vi "traffic lights using parallelism.vi"() -> ()   [LabVIEW 2018]
panel:
  out "GREEN":bool
  out "YELLOW":bool
  out "RED":bool
  out "7 2":bool
  out "6 2":bool
  out "5 2":bool
  out "4 2":bool
  out "3 2":bool
  out "2 2":bool
  out "1 2":bool
  out "7":bool
  out "6":bool
  out "5":bool
  out "4":bool
  out "3":bool
  out "2":bool
  out "1":bool
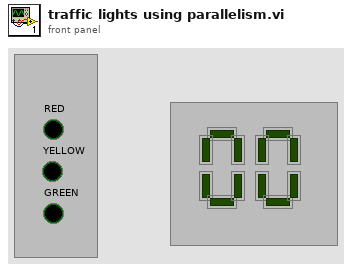
[diagram p1: front panel]
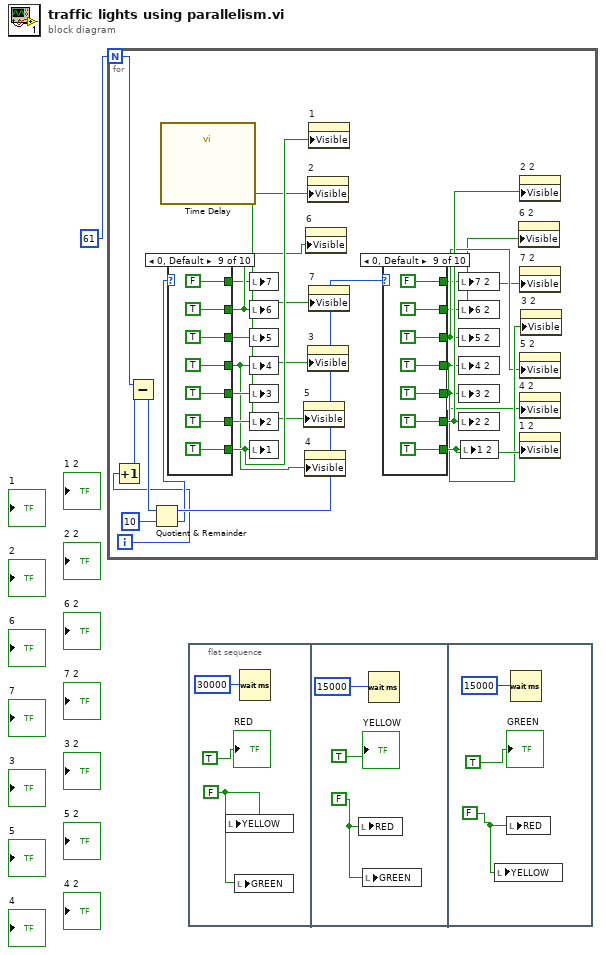
[diagram p0: block diagram]
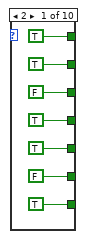
[diagram p2: hidden frame]
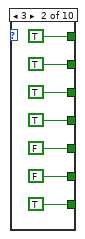
[diagram p3: hidden frame]
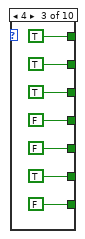
[diagram p4: hidden frame]
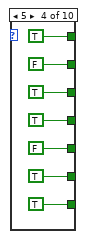
[diagram p5: hidden frame]
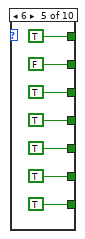
[diagram p6: hidden frame]
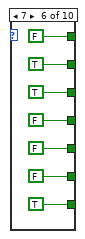
[diagram p7: hidden frame]
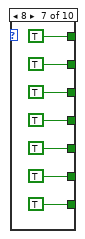
[diagram p8: hidden frame]
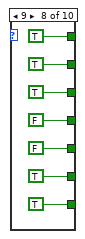
[diagram p9: hidden frame]
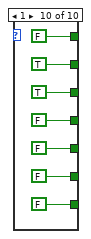
[diagram p10: hidden frame]
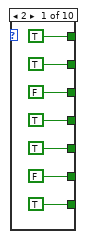
[diagram p11: hidden frame]
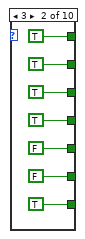
[diagram p12: hidden frame]
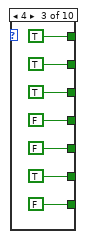
[diagram p13: hidden frame]
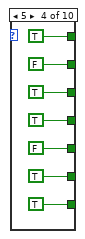
[diagram p14: hidden frame]
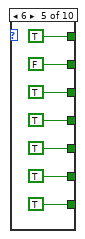
[diagram p15: hidden frame]
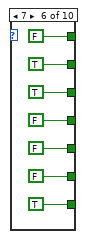
[diagram p16: hidden frame]
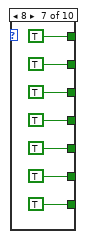
[diagram p17: hidden frame]
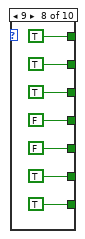
[diagram p18: hidden frame]
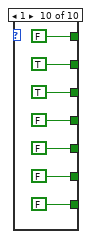
[diagram p19: hidden frame]
diagram:
  n1 = for {
    N: 61 -> [w5]
    i -> [w3]
    n2 = Increment(x=w3) -> (x+1=w2:i32)
    n3 = Subtract(x=w5, y=w2) -> (x-y=w4:i32)
    n4 = Quotient & Remainder(x=w4, y=10) -> (x-y*floor(x/y)=w21:i32, floor(x/y)=w20:i32)
    n5 = call "Time Delay"() -> ()  [unwired: 11 in, 1 out]
    n6 = case shown="0, Default" w20 {
      tunnel: [TRUE TRUE FALSE TRUE TRUE TRUE TRUE TRUE TRUE FALSE] -> w12
      tunnel: [FALSE FALSE TRUE TRUE TRUE FALSE TRUE TRUE TRUE FALSE] -> w11
      tunnel: [TRUE FALSE FALSE FALSE TRUE FALSE TRUE FALSE TRUE FALSE] -> w10
      tunnel: [TRUE TRUE FALSE TRUE TRUE FALSE TRUE FALSE TRUE FALSE] -> w9
      tunnel: [FALSE TRUE TRUE TRUE TRUE TRUE TRUE TRUE TRUE TRUE] -> w8
      tunnel: [TRUE TRUE TRUE FALSE FALSE TRUE TRUE TRUE TRUE TRUE] -> w7
      tunnel: [TRUE TRUE TRUE TRUE TRUE FALSE TRUE TRUE FALSE FALSE] -> w6
      frame 2 {
      }
      frame 3 {
      }
      frame 4 {
      }
      frame 5 {
      }
      frame 6 {
      }
      frame 7 {
      }
      frame 8 {
      }
      frame 9 {
      }
      frame 0, Default {
      }
      frame 1 {
      }
    }
    n7 = local write "7"(w6) -> ()
    n8 = local write "6"(w7) -> ()
    n9 = local write "5"(w8) -> ()
    n10 = local write "4"(w9) -> ()
    n11 = local write "3"(w10) -> ()
    n12 = local write "2"(w11) -> ()
    n13 = local write "1"(w12) -> ()
    n14 = property on="5" class="Bool (strict)"("Visible"=w8) -> ()  [unwired: 2 in, 2 out]
    n15 = property on="4" class="Bool (strict)"("Visible"=w9) -> ()  [unwired: 2 in, 2 out]
    n16 = property on="6" class="Bool (strict)"("Visible"=w7) -> ()  [unwired: 2 in, 2 out]
    n17 = property on="2" class="Bool (strict)"("Visible"=w11) -> ()  [unwired: 2 in, 2 out]
    n18 = property on="3" class="Bool (strict)"("Visible"=w10) -> ()  [unwired: 2 in, 2 out]
    n19 = property on="1" class="Bool (strict)"("Visible"=w12) -> ()  [unwired: 2 in, 2 out]
    n20 = property on="7" class="Bool (strict)"("Visible"=w6) -> ()  [unwired: 2 in, 2 out]
    n21 = case shown="0, Default" w21 {
      tunnel: [TRUE TRUE FALSE TRUE TRUE TRUE TRUE TRUE TRUE FALSE] -> w19
      tunnel: [FALSE FALSE TRUE TRUE TRUE FALSE TRUE TRUE TRUE FALSE] -> w18
      tunnel: [TRUE FALSE FALSE FALSE TRUE FALSE TRUE FALSE TRUE FALSE] -> w17
      tunnel: [TRUE TRUE FALSE TRUE TRUE FALSE TRUE FALSE TRUE FALSE] -> w16
      tunnel: [FALSE TRUE TRUE TRUE TRUE TRUE TRUE TRUE TRUE TRUE] -> w15
      tunnel: [TRUE TRUE TRUE FALSE FALSE TRUE TRUE TRUE TRUE TRUE] -> w14
      tunnel: [TRUE TRUE TRUE TRUE TRUE FALSE TRUE TRUE FALSE FALSE] -> w13
      frame 2 {
      }
      frame 3 {
      }
      frame 4 {
      }
      frame 5 {
      }
      frame 6 {
      }
      frame 7 {
      }
      frame 8 {
      }
      frame 9 {
      }
      frame 0, Default {
      }
      frame 1 {
      }
    }
    n22 = local write "7 2"(w13) -> ()
    n23 = local write "6 2"(w14) -> ()
    n24 = local write "5 2"(w15) -> ()
    n25 = local write "4 2"(w16) -> ()
    n26 = local write "3 2"(w17) -> ()
    n27 = local write "2 2"(w18) -> ()
    n28 = local write "1 2"(w19) -> ()
    n29 = property on="6 2" class="Bool (strict)"("Visible"=w14) -> ()  [unwired: 2 in, 2 out]
    n30 = property on="2 2" class="Bool (strict)"("Visible"=w18) -> ()  [unwired: 2 in, 2 out]
    n31 = property on="7 2" class="Bool (strict)"("Visible"=w13) -> ()  [unwired: 2 in, 2 out]
    n32 = property on="5 2" class="Bool (strict)"("Visible"=w15) -> ()  [unwired: 2 in, 2 out]
    n33 = property on="4 2" class="Bool (strict)"("Visible"=w16) -> ()  [unwired: 2 in, 2 out]
    n34 = property on="1 2" class="Bool (strict)"("Visible"=w19) -> ()  [unwired: 2 in, 2 out]
    n35 = property on="3 2" class="Bool (strict)"("Visible"=w17) -> ()  [unwired: 2 in, 2 out]
  }
  n36 = flat-sequence {
    frame #0 {
      w163 = FALSE ("Boolean")
      n37 = local write "YELLOW"(w163) -> ()
      n38 = local write "GREEN"(w163) -> ()
      n39 = Wait (ms)(milliseconds to wait=u32 30000 ("millisecond timer value")) -> ()  [unwired: 1 out]
      "RED" <- TRUE ("Boolean")
    }
    frame #1 {
      w166 = FALSE ("Boolean")
      n40 = local write "RED"(w166) -> ()
      n41 = local write "GREEN"(w166) -> ()
      n42 = Wait (ms)(milliseconds to wait=u32 15000 ("millisecond timer value")) -> ()  [unwired: 1 out]
      "YELLOW" <- TRUE ("Boolean")
    }
    frame #2 {
      w169 = FALSE ("Boolean")
      n43 = local write "YELLOW"(w169) -> ()
      n44 = local write "RED"(w169) -> ()
      n45 = Wait (ms)(milliseconds to wait=u32 15000 ("millisecond timer value")) -> ()  [unwired: 1 out]
      "GREEN" <- TRUE ("Boolean")
    }
  }
